vi "RT Loop - RSI Control.vi"(11 "Message Queue":refnum<queue>) -> ()   [LabVIEW 2017]
doc: "This RSI Control Loop VI performs control calculations on four input channels in parallel, and outputs the results to four output channels."
uses:
  support/Message Queue/Message Cluster.ctl
  <vilib>/Platform/TimedLoop/XDataNode/timing_clust.ctl
  <vilib>/Platform/TimedLoop/XDataNode/nitl_modes.ctl
  <vilib>/Platform/TimedLoop/XDataNode/wakeup.ctl
  controls/Control State.ctl
  <vilib>/Platform/TimedLoop/XDataNode/loadnilvce.vi
  <vilib>/addons/control/pid/pid.llb/PID (DBL).vi
  <vilib>/Platform/TimedLoop/XDataNode/XDataNode.xnode
  <vilib>/Platform/TimedLoop/XDataNode/XDNodeRunTimeDep.lvlib
  <vilib>/addons/control/pid/NI_PID_pid.lvlib
  support/Message Queue/Message Queue.lvlib
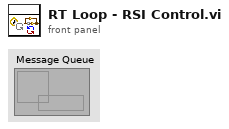
[diagram p1: front panel]
types:
  T1 = typedef "XDNodeRunTimeDep.lvlib/timing_clust.ctl" = cluster{"Expected End [f-1]":u64, "Actual End [f-1]":u64, "Finished Late? [f-1]":bool, "Expected End [i-1]":u64, "Actual End [i-1]":u64, "Finished Late? [i-1]":bool, "Expected Start [i]":u64, "Actual Start [i]":u64, "Expected Start [f]":u64, "Actual Start [f]":u64, "Source Name":string, "Structure Name":string, "Period":i64, "Deadline":i64, "Offset":i64, "Start":i64, "Priority":i32, "Timeout":i32, "Mode":T2, "Wakeup Reason":T3, "Error":errorcluster, "Source Type":string, "Secondary Source Type":string, "Global End Time":u64, "Global Start Time":u64, "Frame Duration":u64, "Iteration Duration":u64, "Assigned CPU":i32, "I/O Scan Engine Mode":u32}
  T2 = typedef "XDNodeRunTimeDep.lvlib/nitl_modes.ctl" = enum32{"No Change", "Process missed periods, maintain original phase", "Discard missed periods, maintain original phase", "Process missed periods, ignore original phase", "Discard missed periods, ignore original phase"}
  T3 = typedef "XDNodeRunTimeDep.lvlib/wakeup.ctl" = enum32{"Normal", "Aborted", "Asynchronous wakeup", "Timing source error", "Timed loop error", "Timeout"}
  T4 = cluster{"static gain":dbl, "lag (s)":dbl, "deadtime (s)":dbl, "load":dbl, "deadband":dbl, "sensor noise":dbl, "initial PV":dbl, "plant noise":dbl}
  T5 = typedef "Control State.ctl" = enum16{"Safe State", "Control (PID)"}
  T6 = typedef "Control Configuration.ctl" = cluster{"PID Gains":cluster{"proportional gain (Kc)":dbl, "integral gain (Kc*Ts/Ti)":dbl, "derivative gain (Kc*Td/Ts)":dbl}, "Output Range":cluster{"output high":dbl, "output low":dbl}}
  T7 = cluster{"proportional gain (Kc)":dbl, "integral gain (Kc*Ts/Ti)":dbl, "derivative gain (Kc*Td/Ts)":dbl}
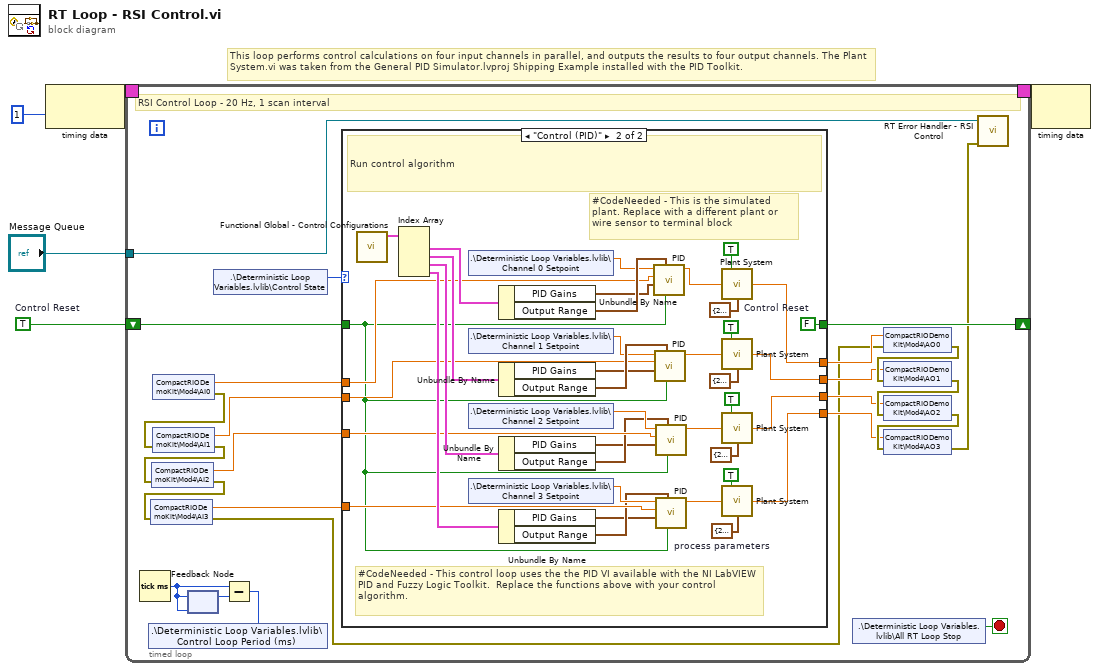
[diagram p0: block diagram]
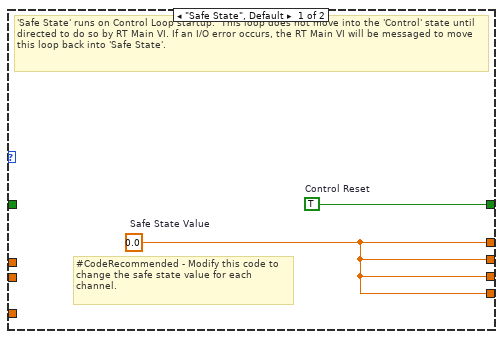
[diagram p2: hidden frame]
diagram:
  w5 = TRUE  # Control Reset
  # "This loop performs control calculations on four input channels in parallel, and outputs the results to four output channels. The Plant System.vi was taken from the General PID Simulator.lvproj Shipping Example installed with the PID Toolkit."
  n1 = node-c288(i64 1 ("Period")) -> (w4:T1)
  n2 = timed-loop {
    shift-right: [w29] -> _
    shift-left: w5 -> [w28]
    timing: w4 -> [_]
    timing-out: [_] -> w3
    tunnel: "Message Queue" -> [w14]
    stop <- w11 stop-if-true
    # "RSI Control Loop - 20 Hz, 1 scan interval"
    n3 = Tick Count (ms)() -> (millisecond timer value=w13:u32)
    n4 = shared-variable "CompactRIODemoKit\\Mod4\\AI0"() -> (w7:dbl, error out=w27:errorcluster)  [unwired: 1 in]
    n5 = shared-variable "CompactRIODemoKit\\Mod4\\AI1"(error in=w27) -> (w24:dbl, error out=w26:errorcluster)
    n6 = shared-variable "CompactRIODemoKit\\Mod4\\AI2"(error in=w26) -> (w6:dbl, error out=w25:errorcluster)
    n7 = shared-variable "CompactRIODemoKit\\Mod4\\AI3"(error in=w25) -> (w8:dbl, error out=w16:errorcluster)
    n8 = feedback-in #1(w13) -> ()
    n9 = feedback #1(w13) -> (w12:u32)
    n10 = shared-variable ".\\Deterministic Loop Variables.lvlib\\Control State"() -> (w9:T5)  [unwired: 1 in, 1 out]
    n11 = Subtract(x=w13, y=w12) -> (x-y=w10:u32)
    n12 = shared-variable ".\\Deterministic Loop Variables.lvlib\\Control Loop Period (ms)"(w10) -> ()  [unwired: 1 in, 1 out]
    n13 = case shown="\"Control (PID)\"" w9 {
      tunnel: w7 -> [_ w61]
      tunnel: [w30 w43] -> w23
      tunnel: [w31 w70] -> w29
      tunnel: w28 -> [_ w48]
      tunnel: w24 -> [_ w57]
      tunnel: w6 -> [_ w56]
      tunnel: w8 -> [_ w52]
      tunnel: [w30 w42] -> w19
      tunnel: [w30 w41] -> w18
      tunnel: [w30 w40] -> w17
      frame "Safe State", Default {
        w30 = 0.0  # Safe State Value
        w31 = TRUE  # Control Reset
        # "#CodeRecommended - Modify this code to change the safe state value for each channel."
        # "'Safe State' runs on Control Loop startup.  This loop does not move into the 'Control' state until directed to do so by RT Main VI. If an I/O error occurs, the RT Main VI will be messaged to move this loop back into 'Safe State'."
      }
      frame "Control (PID)" {
        w35 = T4 {"static gain"=2.5, "lag (s)"=2.5, "deadtime (s)"=0.001, "load"=0.0, "deadband"=0.0, "sensor noise"=0.0, "initial PV"=5.0, "plant noise"=0.0}  # process parameters
        w70 = FALSE  # Control Reset
        # "#CodeNeeded - This is the simulated plant. Replace with a different plant or wire sensor to terminal block"
        # "#CodeNeeded - This control loop uses the the PID VI available with the NI LabVIEW PID and Fuzzy Logic Toolkit.  Replace the functions above with your control algorithm."
        # "Run control algorithm"
        n14 = call "Functional Global - Control Configurations.vi"() -> ("Control Configurations out"=w69:T6[])  [unwired: 11 in]
        n15 = Index Array(array=w69) -> (element #1=w68:T6, element #2=w67:T6, element #3=w66:T6, element #4=w65:T6)  [unwired: 4 in]
        n16 = shared-variable ".\\Deterministic Loop Variables.lvlib\\Channel 0 Setpoint"() -> (w62:dbl)  [unwired: 1 in, 1 out]
        n17 = shared-variable ".\\Deterministic Loop Variables.lvlib\\Channel 1 Setpoint"() -> (w58:dbl)  [unwired: 1 in, 1 out]
        n18 = shared-variable ".\\Deterministic Loop Variables.lvlib\\Channel 2 Setpoint"() -> (w55:dbl)  [unwired: 1 in, 1 out]
        n19 = shared-variable ".\\Deterministic Loop Variables.lvlib\\Channel 3 Setpoint"() -> (w51:dbl)  [unwired: 1 in, 1 out]
        n20 = Unbundle By Name(w68) -> ("PID Gains"=w63:T7, "Output Range"=w64:cluster{"output high":dbl, "output low":dbl})
        n21 = Unbundle By Name(w67) -> ("PID Gains"=w59:T7, "Output Range"=w60:cluster{"output high":dbl, "output low":dbl})
        n22 = Unbundle By Name(w66) -> ("PID Gains"=w53:T7, "Output Range"=w54:cluster{"output high":dbl, "output low":dbl})
        n23 = Unbundle By Name(w65) -> ("PID Gains"=w49:T7, "Output Range"=w50:cluster{"output high":dbl, "output low":dbl})
        n24 = call-poly <vilib>:"PID.vi"("reinitialize? (F)"=w48, "output range"=w64, "PID gains"=w63, "process variable"=w61, "setpoint"=w62) -> ("output"=w44:dbl)  [unwired: 5 in, 1 out]
        n25 = call-poly <vilib>:"PID.vi"("reinitialize? (F)"=w48, "output range"=w60, "PID gains"=w59, "process variable"=w57, "setpoint"=w58) -> ("output"=w45:dbl)  [unwired: 5 in, 1 out]
        n26 = call-poly <vilib>:"PID.vi"("reinitialize? (F)"=w48, "output range"=w54, "PID gains"=w53, "process variable"=w56, "setpoint"=w55) -> ("output"=w46:dbl)  [unwired: 5 in, 1 out]
        n27 = call-poly <vilib>:"PID.vi"("reinitialize? (F)"=w48, "output range"=w50, "PID gains"=w49, "process variable"=w52, "setpoint"=w51) -> ("output"=w47:dbl)  [unwired: 5 in, 1 out]
        n28 = call "Plant System.vi"("Integrator?"=TRUE, "Plant Input"=w44, "process parameters"=T4 {"static gain"=2.5, "lag (s)"=2.5, "deadtime (s)"=0.001, "load"=0.0, "deadband"=0.0, "sensor noise"=0.0, "initial PV"=5.0, "plant noise"=0.0}) -> ("Plant Output"=w43:dbl)  [unwired: 12 in]
        n29 = call "Plant System.vi"("Integrator?"=TRUE, "Plant Input"=w45, "process parameters"=T4 {"static gain"=2.5, "lag (s)"=2.5, "deadtime (s)"=0.001, "load"=0.0, "deadband"=0.0, "sensor noise"=0.0, "initial PV"=5.0, "plant noise"=0.0}) -> ("Plant Output"=w42:dbl)  [unwired: 12 in]
        n30 = call "Plant System.vi"("Integrator?"=TRUE, "Plant Input"=w46, "process parameters"=T4 {"static gain"=2.5, "lag (s)"=2.5, "deadtime (s)"=0.001, "load"=0.0, "deadband"=0.0, "sensor noise"=0.0, "initial PV"=5.0, "plant noise"=0.0}) -> ("Plant Output"=w41:dbl)  [unwired: 12 in]
        n31 = call "Plant System.vi"("Integrator?"=TRUE, "Plant Input"=w47, "process parameters"=w35) -> ("Plant Output"=w40:dbl)  [unwired: 12 in]
      }
    }
    n32 = shared-variable ".\\Deterministic Loop Variables.lvlib\\All RT Loop Stop"() -> (w11:bool)  [unwired: 1 in, 1 out]
    n33 = shared-variable "CompactRIODemoKit\\Mod4\\AO0"(w23, error in=w16) -> (error out=w22:errorcluster)
    n34 = shared-variable "CompactRIODemoKit\\Mod4\\AO1"(w19, error in=w22) -> (error out=w21:errorcluster)
    n35 = shared-variable "CompactRIODemoKit\\Mod4\\AO2"(w18, error in=w21) -> (error out=w20:errorcluster)
    n36 = shared-variable "CompactRIODemoKit\\Mod4\\AO3"(w17, error in=w20) -> (error out=w15:errorcluster)
    n37 = call "RT Error Handler - RSI Control.vi"("error in (no error)"=w15, "Message Queue"=w14) -> ()  [unwired: 8 in, 2 out]
  }
  n38 = node-c288(w3) -> ()  [unwired: 1 out]
